vi "Launcher.vi"() -> ()   [LabVIEW 2014]
uses:
  Launcher-state.ctl
panel:
  out "Count":dbl
  in  "Launch":bool
  in  "Abort":bool
  out "Engines":bool
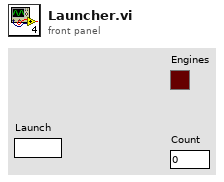
[diagram p1: front panel]
types:
  T1 = typedef "Launcher-state.ctl" = enum16{"Ready", "CountDown", "Fire", "EngineStop", "Abort"}
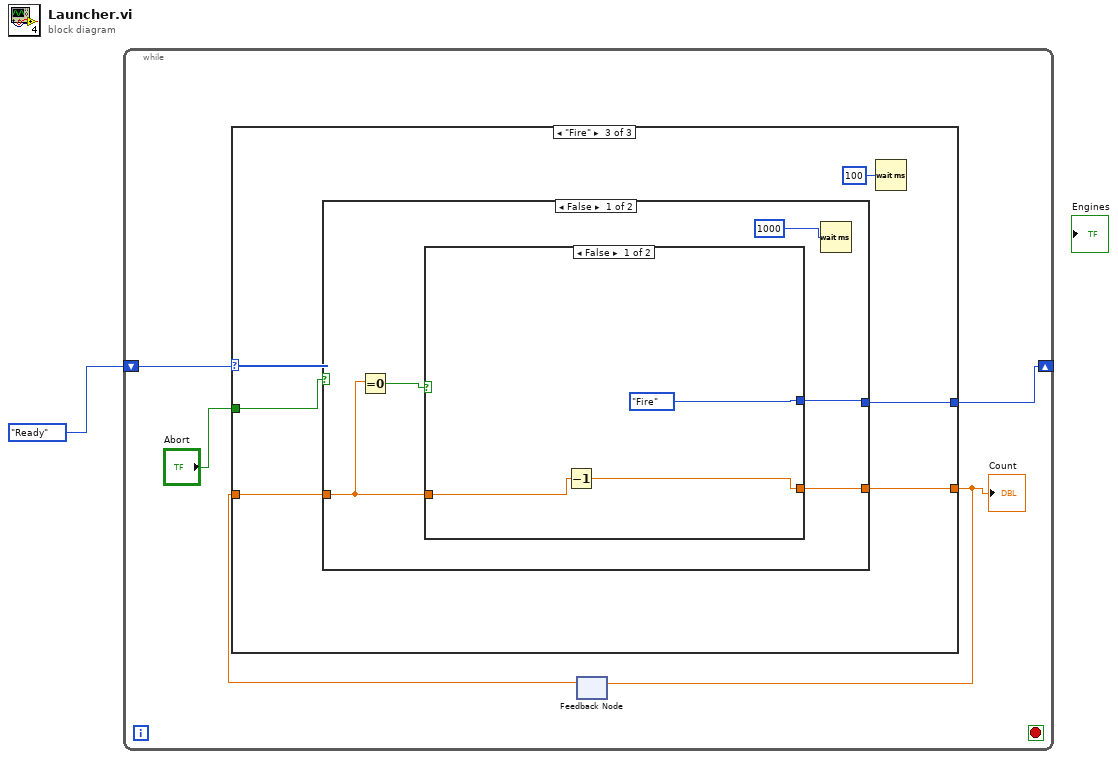
[diagram p0: block diagram]
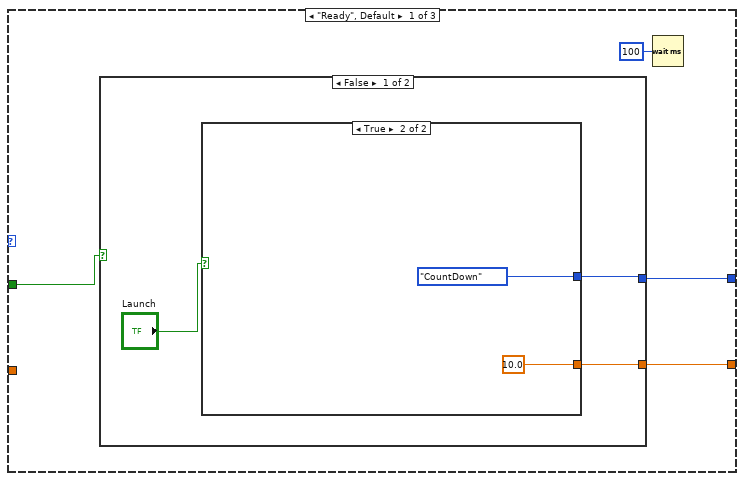
[diagram p2: hidden frame]
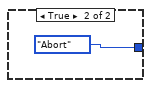
[diagram p4: hidden frame]
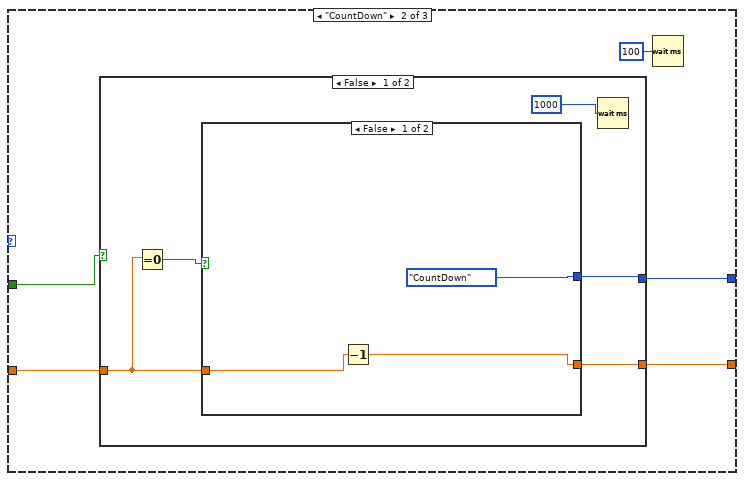
[diagram p5: hidden frame]
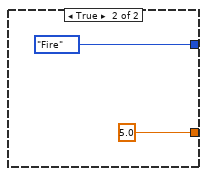
[diagram p6: hidden frame]
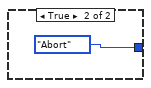
[diagram p7: hidden frame]
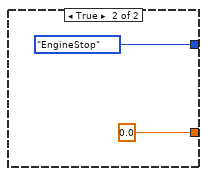
[diagram p8: hidden frame]
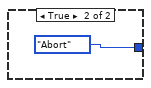
[diagram p9: hidden frame]
diagram:
  n1 = while {
    shift-right: [w5] -> _
    shift-left: Launcher-state."Ready" ("Launch State") -> [w6]
    stop <- _ stop-if-true
    n2 = feedback #1() -> (w2:dbl)  [unwired: 1 in]
    n3 = case shown="\"Fire\"" w6 {
      tunnel: [w10 w21 w37] -> w5
      tunnel: "Abort" -> [w9 w20 w36]
      tunnel: [w7 w18 w34] -> w3
      tunnel: w2 -> [_ w17 w33]
      frame "Ready", Default {
        n4 = case shown="False" w9 {
          tunnel: [w11 Launcher-state."Abort" ("Launch State")] -> w10
          tunnel: [w13 _] -> w7
          frame False {
            n5 = case shown="True" "Launch" {
              tunnel: [_ 10.0] -> w13
              tunnel: [_ Launcher-state."CountDown" ("Launch State")] -> w11
              frame False {
              }
              frame True {
              }
            }
          }
          frame True {
          }
        }
        n6 = Wait (ms)(milliseconds to wait=u32 100) -> ()  [unwired: 1 out]
      }
      frame "CountDown" {
        n7 = case shown="False" w20 {
          tunnel: [w25 Launcher-state."Abort" ("Launch State")] -> w21
          tunnel: [w26 _] -> w18
          tunnel: w17 -> [w24 _]
          frame False {
            n8 = Equal To 0?(x=w24) -> (x = 0?=w23:bool)
            n9 = case shown="False" w23 {
              tunnel: [w28 5.0] -> w26
              tunnel: [Launcher-state."CountDown" ("Launch State") Launcher-state."Fire" ("Launch State")] -> w25
              tunnel: w24 -> [w29 _]
              frame False {
                n10 = Decrement(x=w29) -> (x-1=w28:dbl)
              }
              frame True {
              }
            }
            n11 = Wait (ms)(milliseconds to wait=u32 1000) -> ()  [unwired: 1 out]
          }
          frame True {
          }
        }
        n12 = Wait (ms)(milliseconds to wait=u32 100) -> ()  [unwired: 1 out]
      }
      frame "Fire" {
        n13 = case shown="False" w36 {
          tunnel: [w41 Launcher-state."Abort" ("Launch State")] -> w37
          tunnel: [w42 _] -> w34
          tunnel: w33 -> [w40 _]
          frame False {
            n14 = Equal To 0?(x=w40) -> (x = 0?=w39:bool)
            n15 = case shown="False" w39 {
              tunnel: [w44 0.0] -> w42
              tunnel: [Launcher-state."Fire" ("Launch State") Launcher-state."EngineStop" ("Launch State")] -> w41
              tunnel: w40 -> [w45 _]
              frame False {
                n16 = Decrement(x=w45) -> (x-1=w44:dbl)
              }
              frame True {
              }
            }
            n17 = Wait (ms)(milliseconds to wait=u32 1000) -> ()  [unwired: 1 out]
          }
          frame True {
          }
        }
        n18 = Wait (ms)(milliseconds to wait=u32 100) -> ()  [unwired: 1 out]
      }
    }
    "Count" <- w3
    n19 = feedback-in #1(w3) -> ()
  }
